vi "Reset.vi"(8 "error in (no error)":errorcluster, 11 "session in":T1) -> (0 "error out":errorcluster, 3 "session out":T1)   [LabVIEW 2020, in "SLSC Switch.lvlib"]
doc: "Disconnects all created paths and returns the switch module to the state at initialization."
uses:
  <vilib>/SLSC_Switch/SLSC Switch.lvlib
  nislscsl.dll
  <vilib>/userdefined/High Color/SLSC_Switch/nislscslSession.ctl
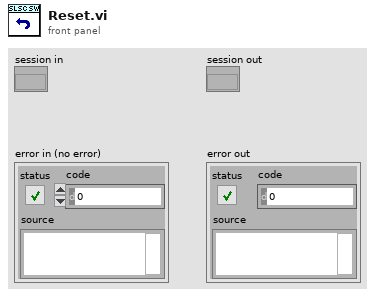
[diagram p1: front panel]
types:
  T1 = typedef "nislscslSession.ctl" = refnum<k20>
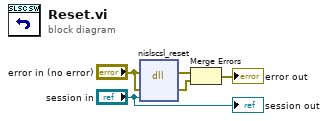
[diagram p0: block diagram]
diagram:
  n1 = dll-call lib="nislscsl.*" fn="nislscsl_reset"(error in="error in (no error)", "errorCluster"="error in (no error)", "sessionHandle"="session in") -> (error out=w5:errorcluster, "errorCluster"=w4:errorcluster)  [unwired: 4 in, 1 out]
  n2 = Merge Errors(w5, w4) -> (→"error out":errorcluster)
  "session out" <- "session in"
